vi "Read Freq Amp Array.vi"(8 "error in (no error)":errorcluster, 11 "Frequency Measurement in":refnum<class "Frequency Measurement.lvclass">) -> (0 "error out":errorcluster, 2 "Freq Amp Array":dbl[][](array[numeric])=[[1000.0, 25750.0, 50500.0, 75250.0, 100000.0], [6.881057614454697, 0.7762788757172112, 3.877116497313211, 5.5398055148465115, 8.936592894514183]], 3 "Frequency Measurement out":refnum<class "Frequency Measurement.lvclass">)   [LabVIEW 2013, in "Frequency Measurement.lvlib" / "Frequency Measurement.lvclass"]
uses:
  Frequency Measurement.lvclass
  Frequency Measurement.lvclass/Frequency Measurement.ctl
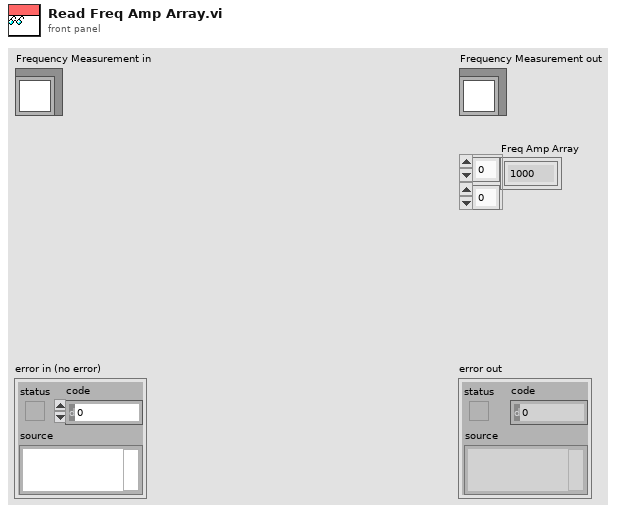
[diagram p1: front panel]
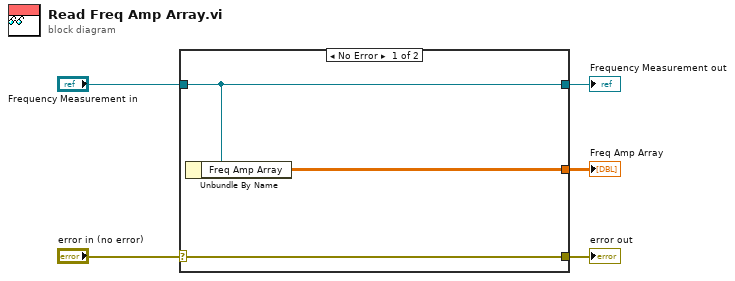
[diagram p0: block diagram]
diagram:
  n1 = case shown="No Error" "error in (no error)" {
    selector: "error in (no error)" -> [w8 w9]
    tunnel: [w8 w9] -> w4
    tunnel: [w7 w10] -> w2
    tunnel: "Frequency Measurement in" -> [w7 w10]
    tunnel: [w6 _] -> w1
    frame No Error {
      n2 = Unbundle By Name(w7) -> ("Freq Amp Array"=w6:dbl[][])
    }
    frame Error {
    }
  }
  "error out" <- w4
  "Frequency Measurement out" <- w2
  "Freq Amp Array" <- w1
